vi "Get Station Config.vi"(8 "error in":errorcluster) -> (0 "error out":errorcluster, 3 "Station Config":T1)   [LabVIEW 2025, in "Full User Interface.lvlib"]
uses:
  Full User Interface.lvlib
  Station Config.ctl
  Station Info.ctl
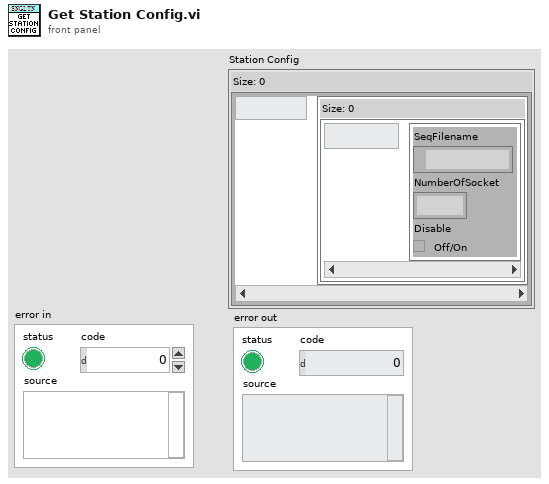
[diagram p1: front panel]
types:
  T1 = typedef "Full User Interface.lvlib/Station Config.ctl" = map{string, map{i32, T2}}
  T2 = typedef "Full User Interface.lvlib/Station Info.ctl" = cluster{"SeqFilename":path, "NumberOfSocket":i32, "Disable":bool}
  T3 = enum16{"open", "replace", "create", "open or create", "replace or create", "replace or create with confirmation"}
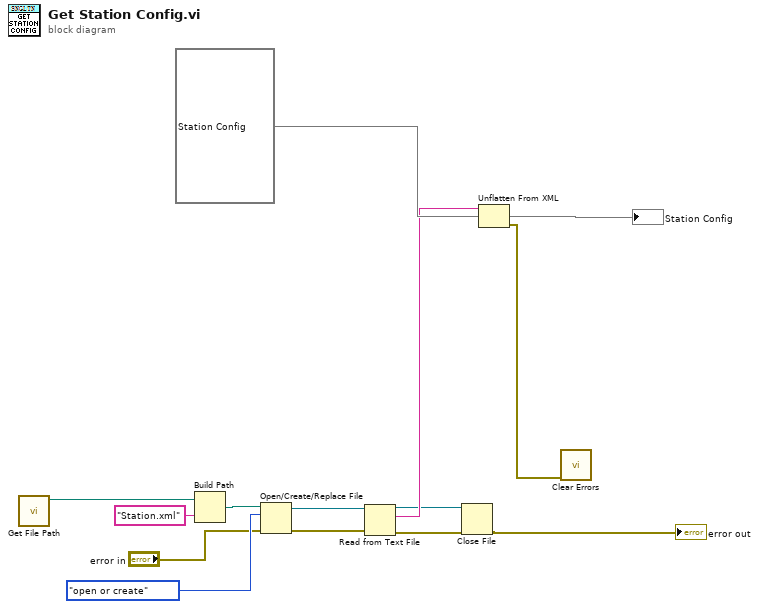
[diagram p0: block diagram]
diagram:
  n1 = call "Get File Path.vi"() -> ("Application Directory"=w8:path)  [unwired: 11 in]
  n2 = Build Path(base path=w8, name or relative path="Station.xml") -> (appended path=w6:path)
  n3 = Open/Create/Replace File(file path (use dialog)=w6, error in="error in", operation (0:open)=T3."open or create") -> (refnum out=w13:refnum<file>, error out=w12:errorcluster)  [unwired: 3 in, 1 out]
  n4 = Read from Text File(file (use dialog)=w13, error in=w12) -> (refnum out=w10:refnum<file>, text=w11:string, error out=w9:errorcluster)  [unwired: 2 in, 1 out]
  n5 = Close File(refnum=w10, error in=w9) -> (error out=→"error out":errorcluster)  [unwired: 1 out]
  n6 = Unflatten From XML(xml string=w11, type=T1 {} ("map")) -> (value=→"Station Config":T1, error out=w2:errorcluster)  [unwired: 1 in]
  n7 = call <vilib>:"Clear Errors.vi"("error in (no error)"=w2) -> ()  [unwired: 5 in, 2 out]
